vi "Remove Alias.vi"(8 "error in":errorcluster, 10 "alias":string, 11 "endpoint aliases in":T1 format="%.0x") -> (0 "error out":errorcluster, 3 "endpoint aliases out":T1 format="%.0x")   [LabVIEW 2017, in "Routing and Faulting Scripting.lvlib"]
doc: "Removes the specified alias from the custom device."
uses:
  Routing and Faulting Scripting.lvlib
  <vilib>/NI Veristand/Custom Device API/Custom Device Item Ref.ctl
  <vilib>/NI Veristand/Custom Device API/Custom Device API.lvlib
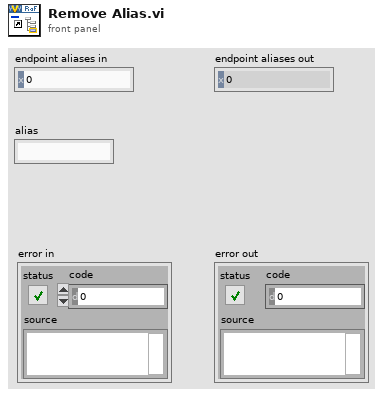
[diagram p1: front panel]
types:
  T1 = typedef "Custom Device API.lvlib/Custom Device Item Ref.ctl" = u64
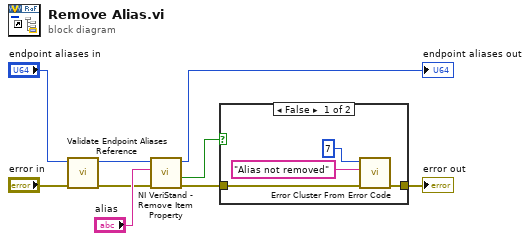
[diagram p0: block diagram]
diagram:
  n1 = call "Validate Endpoint Aliases Reference.vi"("error in"="error in", "endpoint aliases in"="endpoint aliases in") -> ("error out"=w3:errorcluster, "endpoint aliases out"=w1:T1)  [unwired: 8 in]
  n2 = call <vilib>:"NI VeriStand - Remove Item Property.vi"("error in (no error)"=w3, "Property Name"="alias", "Item Ref in"=w1) -> ("error out"=w5:errorcluster, "Removed"=w6:bool, "Item Ref out"=→"endpoint aliases out":T1)  [unwired: 6 in]
  n3 = case shown="False" w6 {
    tunnel: w5 -> [w11 w14]
    tunnel: [w10 w14] -> w4
    frame False {
      n4 = call <vilib>:"Error Cluster From Error Code.vi"("error in (no error)"=w11, "error message (\"\")"="Alias not removed" ("error message (\"\")"), "error code (0)"=7) -> ("error out"=w10:errorcluster)  [unwired: 6 in]
    }
    frame True {
    }
  }
  "error out" <- w4
